vi "ADI_IMU_ADIS16448_Get Instant.vi"(8 "error in":errorcluster, 11 "ADI IMU DevRef":T1={"DevStatus"={"status"=FALSE, "code"=0, "source"=""}, "Handle"=27, "SPI Bus"=enum."SPI MXP", "Device Found"=TRUE, "Device Ready"=FALSE, "Yaw Axis"=enum."Z", "AHRS Algorithm"=enum."Complementary", "Serial"=118, "Lot ID 2"=5379, "Lot ID 1"=118, "Bytes Per Sample"=0, "Calibrate On Open?"=FALSE}) -> (0 "error out":errorcluster, 1 "Sensor Ready Out":bool, 2 "IMU Data Out":T3, 3 "ADI IMU DevRef Out":T1={"DevStatus"={"status"=FALSE, "code"=0, "source"=""}, "Handle"=27, "SPI Bus"=enum."SPI MXP", "Device Found"=TRUE, "Device Ready"=FALSE, "Yaw Axis"=enum."Z", "AHRS Algorithm"=enum."Complementary", "Serial"=118, "Lot ID 2"=5379, "Lot ID 1"=118, "Bytes Per Sample"=0, "Calibrate On Open?"=FALSE})   [LabVIEW 2019, in "ADIS16448_IMU.lvlib"]
doc: "Get instantaneous readings from the Analog Devices MXP IMU board (Gyro Rate, Accel, Magnetometer, Barometer, Temp). This requires that the IMU_Loop VI be located in Periodic Tasks."
uses:
  ADIS16448_IMU.lvlib
  ADI_IMU_ADIS16448_IMUDevRef.ctl
  <vilib>/Rock Robotics/SystemInterfaces/spilib/spi_bus.ctl
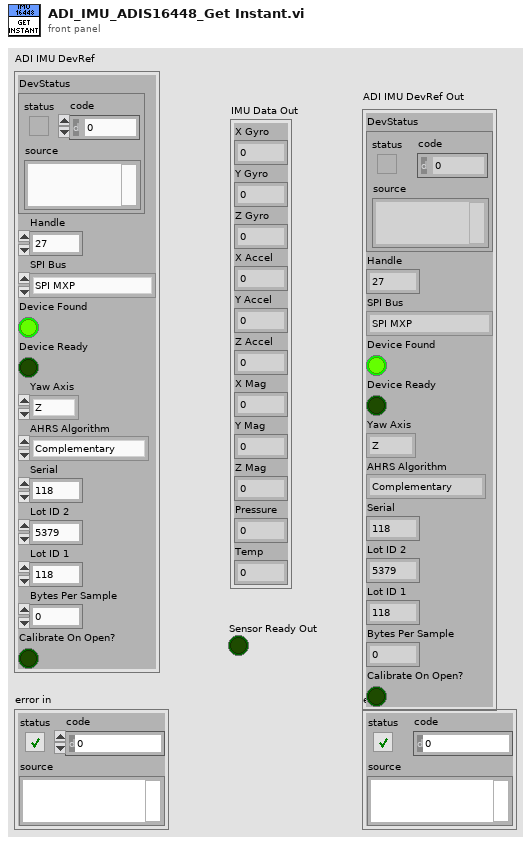
[diagram p1: front panel]
types:
  T1 = typedef "ADIS16448_IMU.lvlib/ADI_IMU_ADIS16448_IMUDevRef.ctl" = cluster{"DevStatus":errorcluster, "Handle":i32, "SPI Bus":T2, "Device Found":bool, "Device Ready":bool, "Yaw Axis":enum16{"X", "Y", "Z"}, "AHRS Algorithm":enum16{"Complementary", "Madgwick"}, "Serial":u16, "Lot ID 2":u16, "Lot ID 1":u16, "Bytes Per Sample":u16, "Calibrate On Open?":bool}
  T2 = typedef "spi_bus.ctl" = enum16{"SPI On-Board, CS0", "SPI On-Board, CS1", "SPI On-Board, CS2", "SPI On-Board, CS3", "SPI MXP", "Invalid"}
  T3 = cluster{"X Gyro":dbl, "Y Gyro":dbl, "Z Gyro":dbl, "X Accel":dbl, "Y Accel":dbl, "Z Accel":dbl, "X Mag":dbl, "Y Mag":dbl, "Z Mag":dbl, "Pressure":dbl, "Temp":dbl}
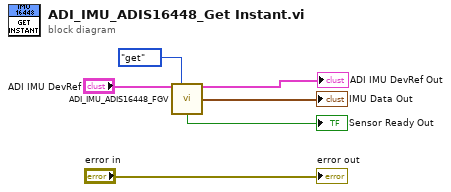
[diagram p0: block diagram]
diagram:
  n1 = call "ADI_IMU_ADIS16448_FGV.vi"("ADI IMU DevRef"="ADI IMU DevRef", "Operation"=enum16{"set", "get", "set reset"}."get") -> ("ADI IMU DevRef Out"=→"ADI IMU DevRef Out":T1, "IMU Data Out"=→"IMU Data Out":T3, "Sensor Ready Out"=→"Sensor Ready Out":bool)  [unwired: 7 in, 4 out]
  "error out" <- "error in"
